vi "K-R.vi"(1 "Град K":dbl) -> (0 "Град R":dbl)   [LabVIEW 2020]
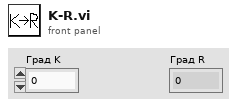
[diagram p1: front panel]
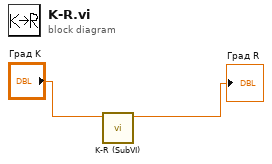
[diagram p0: block diagram]
diagram:
  n1 = call "K-R (SubVI).vi"("Град K"="Град K") -> ("Град R"=→"Град R":dbl)  [unwired: 10 in]
